vi "LOG Update.vi"(8 "error in (no error)":errorcluster, 10 "Message Data":variant, 11 "Data Cluster":T1) -> (0 "error out":errorcluster, 3 "Data Cluster out":T1)   [LabVIEW 2020, in "LOG.lvlib"]
uses:
  LOG.lvlib
  LOG Configuration.ctl
  support/Message Queue/Message Cluster.ctl
  support/Message Queue/Message Queue.lvlib
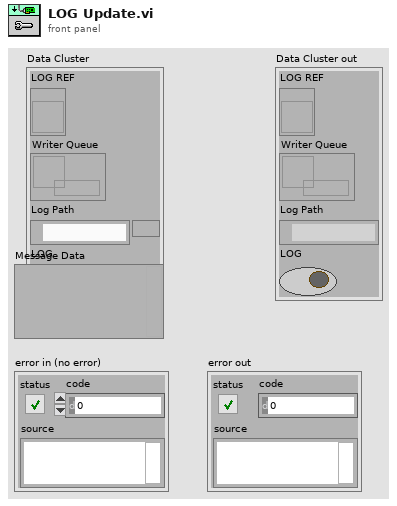
[diagram p1: front panel]
types:
  T1 = typedef "LOG.lvlib/LOG Configuration.ctl" = cluster{"LOG REF":refnum<vi>, "Writer Queue":refnum<queue>, "Log Path":path, "LOG":bool}
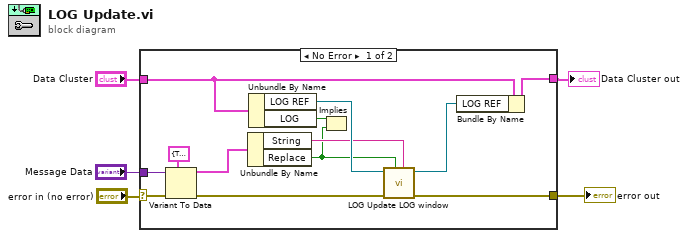
[diagram p0: block diagram]
diagram:
  n1 = case shown="No Error" "error in (no error)" {
    selector: "error in (no error)" -> [w16 w19]
    tunnel: [w18 w20] -> w4
    tunnel: "Data Cluster" -> [w17 w20]
    tunnel: [w11 w19] -> w3
    tunnel: "Message Data" -> [w8 _]
    frame No Error {
      n2 = Variant To Data(error in=w16, type=cluster{"Replace":bool, "String":string} {"Replace"=TRUE, "String"="1"}, Variant=w8) -> (data=w15:cluster{"Replace":bool, "String":string}, error out=w12:errorcluster)
      n3 = Unbundle By Name(w15) -> ("String"=w9:string, "Replace"=w6:bool)
      n4 = Unbundle By Name(w17) -> ("LOG REF"=w14:refnum<vi>, "LOG"=w7:bool)
      n5 = Implies(1:w6, 2:w7) -> ()  [unwired: 1 out]
      n6 = call "LOG Update LOG window.vi"("String"=w9, "replace"=w6, "error in (no error)"=w12, "strLOG in"=w14) -> ("error out"=w11:errorcluster, "strLOG out"=w13:refnum<vi>)  [unwired: 6 in]
      n7 = Bundle By Name(cluster=w17, "LOG REF"=w13) -> (w18:T1)
    }
    frame Error {
    }
  }
  "error out" <- w3
  "Data Cluster out" <- w4
